vi "Work Paper No Record.vi"(8 "error in (no error)":errorcluster, 10 "Work No":refnum<vi>, 11 "Main Process Class in":refnum<class "Main Class.lvclass">) -> (0 "error out":errorcluster, 3 "Main Process Class out":refnum<class "Main Class.lvclass">)   [LabVIEW 2019]
uses:
  Main Class.lvclass
  Ctrl/Table Save.ctl
  LLB/Commonly VI/Main Glb.vi
  <vilib>/Utility/xml.llb/Write to XML File(string).vi
  LLB/Commonly VI.lvlib
panel:
  in  "Boolean":bool
  in  "Work No":string caption="工單號碼"
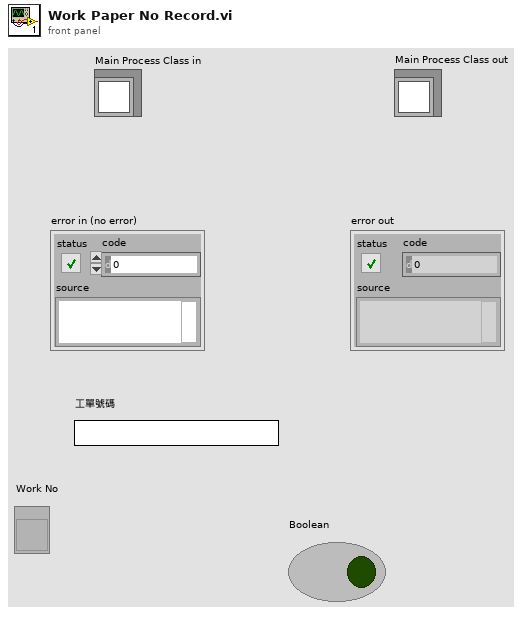
[diagram p1: front panel]
types:
  T1 = cluster{"AutoRunFlg":refnum<vi>, "Action Finish Flg":refnum<vi>, "Remaining Action":refnum<vi>, "Btn_AutoRun":refnum<vi>, "Manual Flg":refnum<vi>, "Sub Process Error":refnum<vi>}
  T2 = typedef "Table Save.ctl" = enum16{"initial", "Add", "Write", "Replace", "Delete", "REad", "RedTable", "Load"}
  T3 = typedef "工單號碼_Index.ctl" = enum16{"工單號碼", "產品料號", "品名", "作業員", "生產總數", "量品數量", "NG數量", "良率%"}
  T4 = cluster{"Work No":string, "產品料號":string, "品名":string, "Operator":string, "工單生產總數":string, "良品出料數量":string, "NG排出數量":string, "Total良率":string}
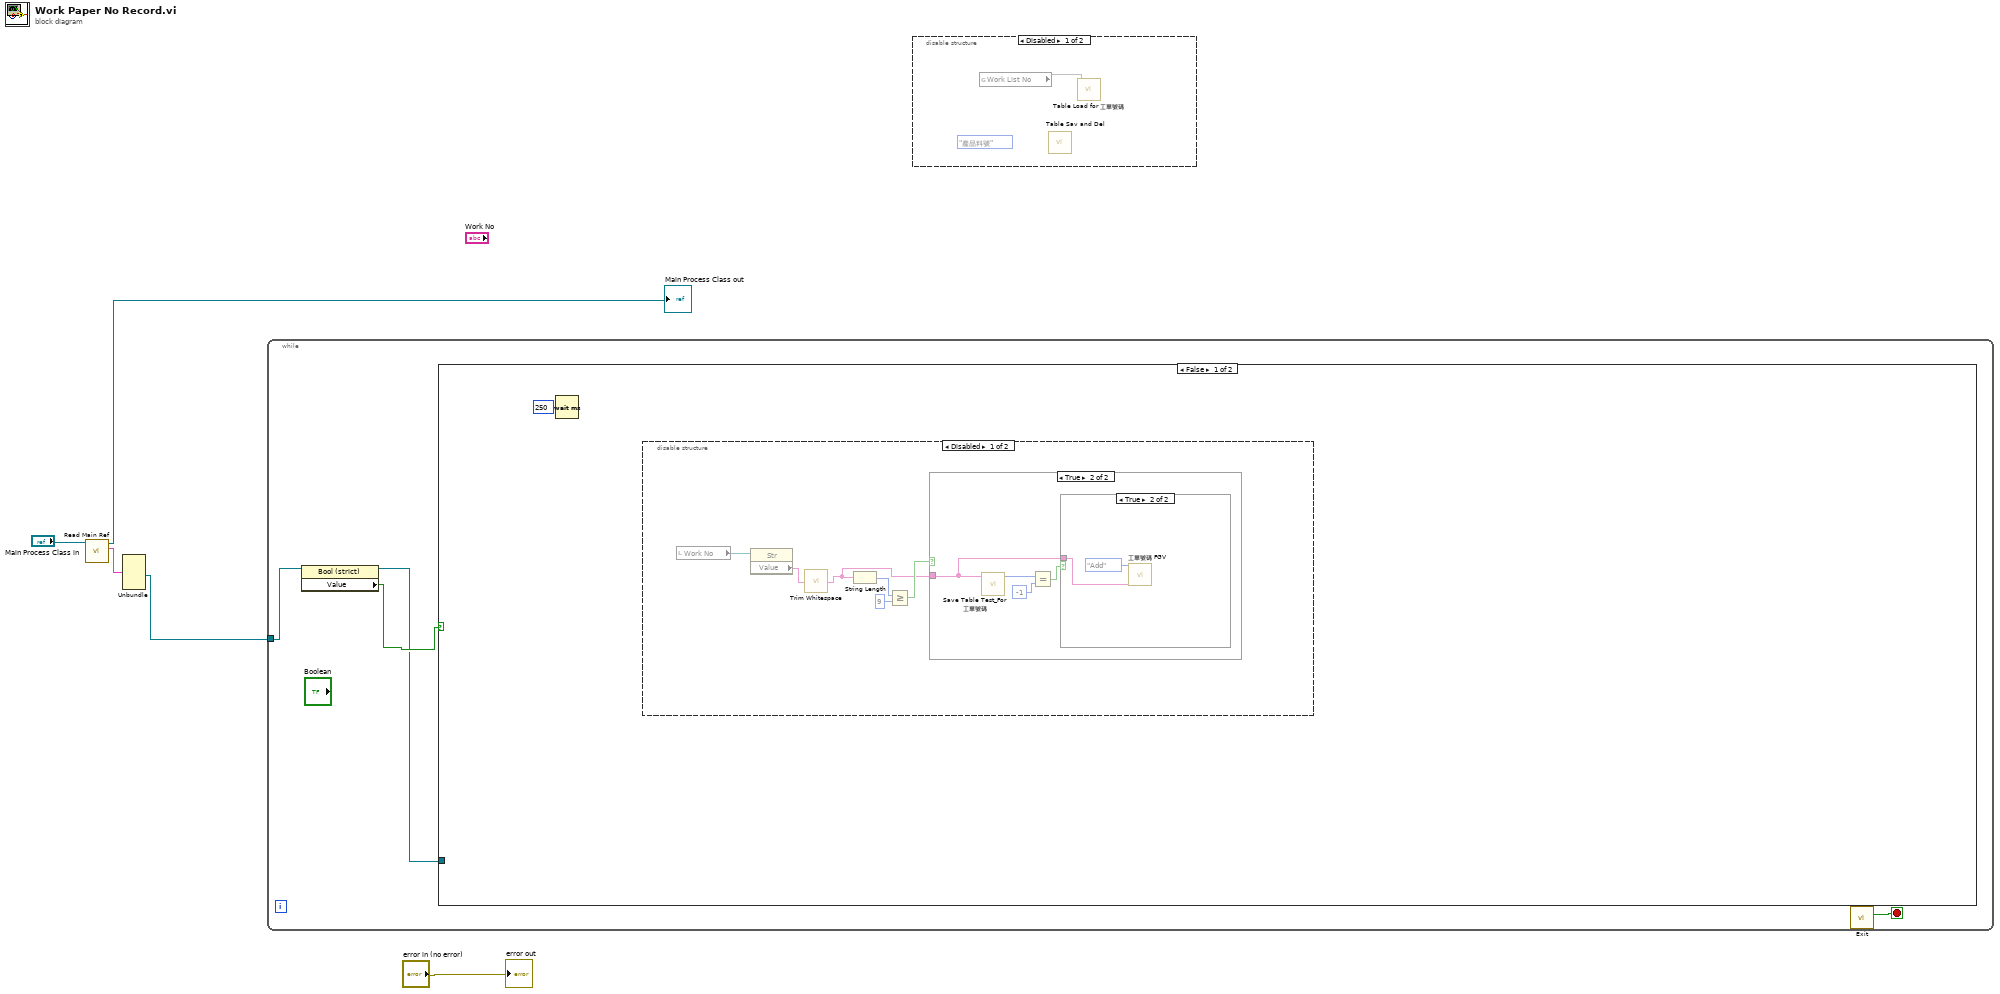
[diagram p0: block diagram]
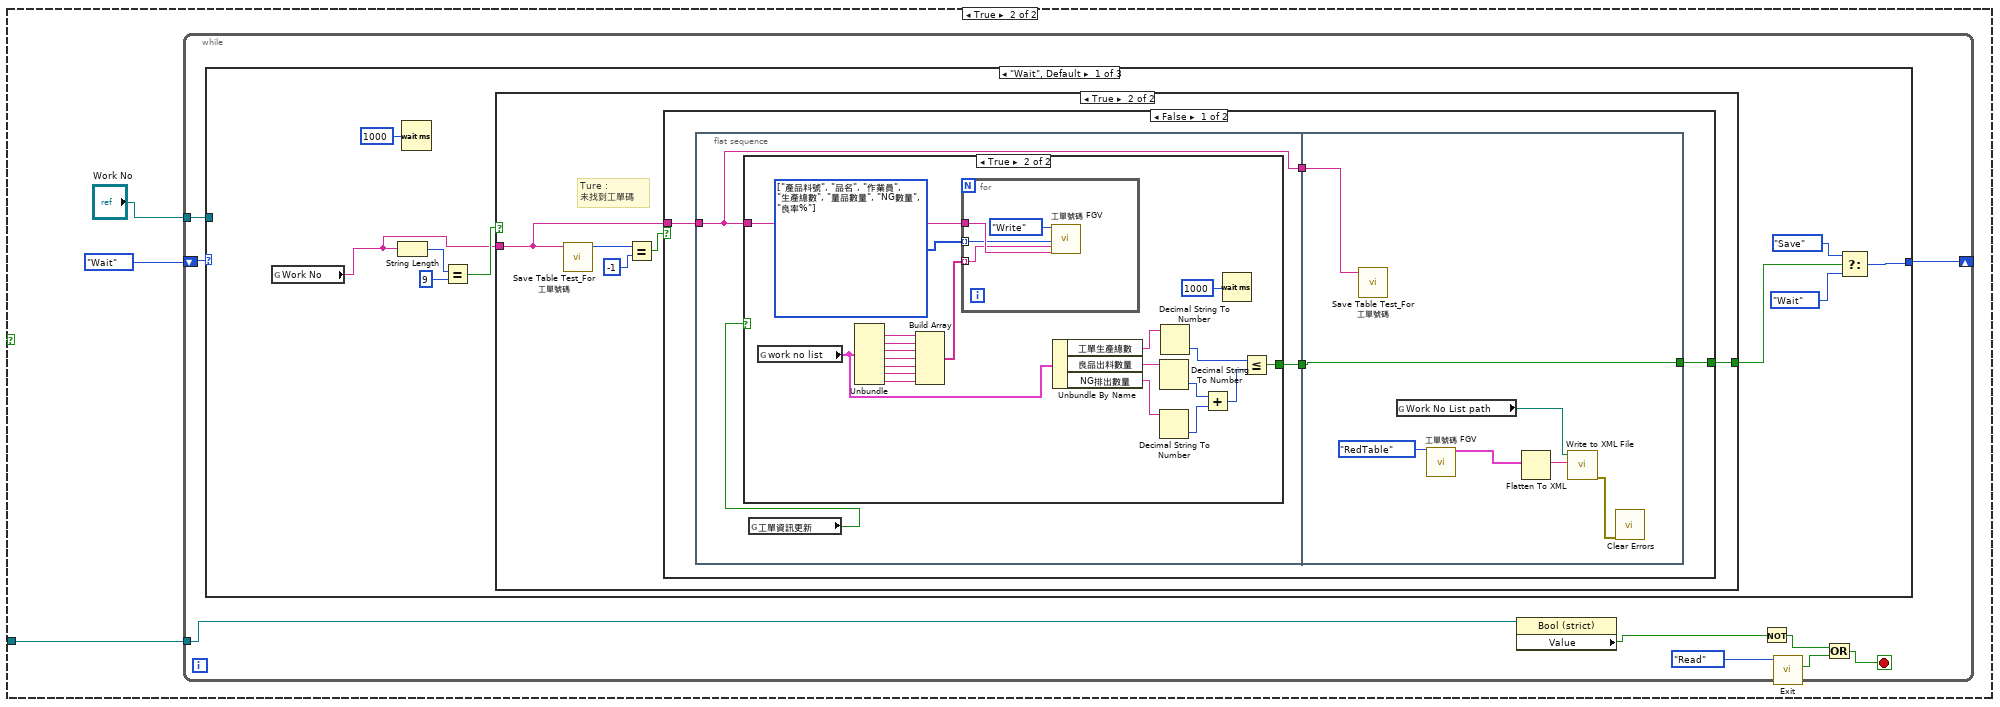
[diagram p6: hidden frame]
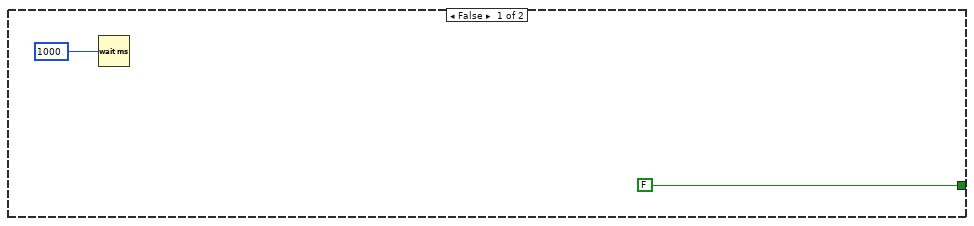
[diagram p7: hidden frame]
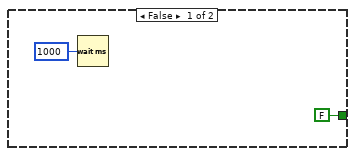
[diagram p8: hidden frame]
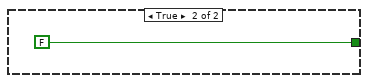
[diagram p9: hidden frame]
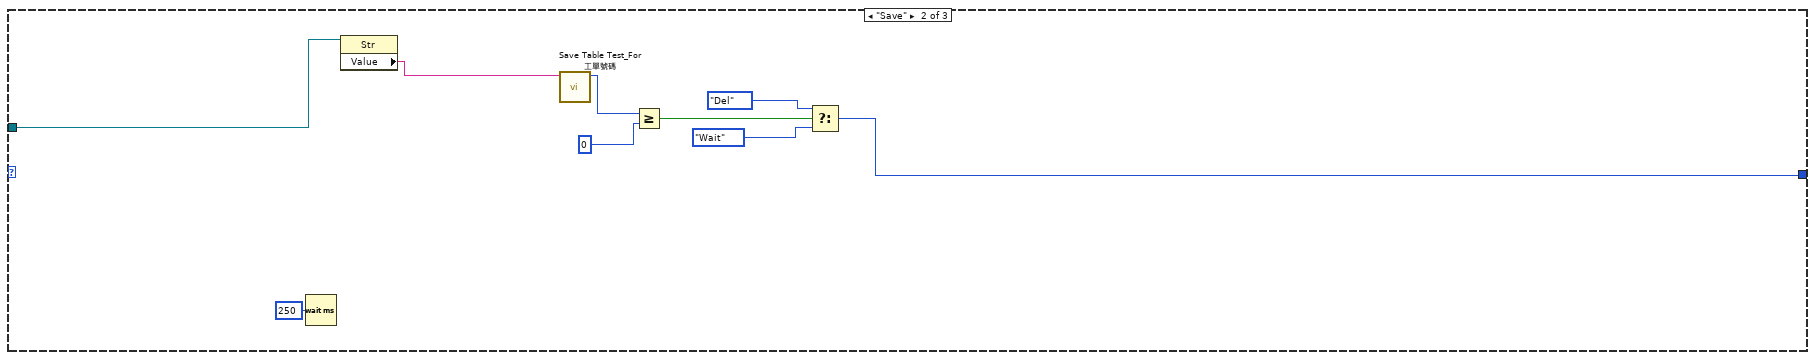
[diagram p10: hidden frame]
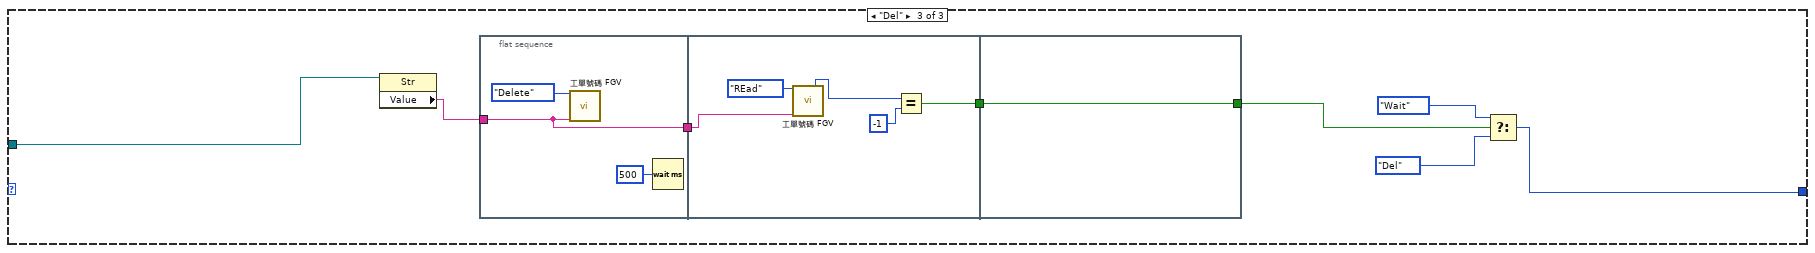
[diagram p11: hidden frame]
diagram:
  n1 = call-dynamic "Read Main Ref.vi"("Main Process Class in"="Main Process Class in") -> ("Main Ref"=w5:T1, "Main Process Class out"=→"Main Process Class out":refnum<class "Main Class.lvclass">)  [unwired: 8 in, 1 out]
  n2 = Unbundle(w5) -> ("Btn_AutoRun"=w2:refnum<vi>)  [unwired: 5 out]
  n3 = while {
    tunnel: w2 -> [w8]
    stop <- w9 stop-if-true
    n4 = property class="Bool (strict)"(reference=w8) -> (reference out=w6:refnum<vi>, "Value"=w7:bool)  [unwired: 1 in, 1 out]
    n5 = case shown="False" w7 {
      tunnel: w6 -> [_ w23]
      frame False {
        n6 = Wait (ms)(milliseconds to wait=u32 250) -> ()  [unwired: 1 out]
        n7 = disable-structure shown="Disabled" {
          frame Disabled {
            n8 = local read "Work No"() -> (w13:refnum<vi>)
            n9 = property class="Str"(reference=w13) -> ("Value"=w12:string)  [unwired: 1 in, 2 out]
            n10 = call <vilib>:"Trim Whitespace.vi"("string"=w12) -> ("trimmed string"=w11:string)  [unwired: 1 in]
            n11 = String Length(string=w11) -> (length=w16:i32)
            n12 = Greater Or Equal?(x=w16, y=9) -> (x >= y?=w14:bool)
            n13 = case shown="True" w14 {
              tunnel: w11 -> [_ w18]
              frame False {
              }
              frame True {
                n14 = call "Save Table Test_For 工單號碼.vi"("工單號碼"=w18) -> ("條碼的Index"=w19:i32)  [unwired: 9 in, 1 out]
                n15 = Equal?(x=w19, y=-1) -> (x = y?=w17:bool)
                n16 = case shown="True" w17 {
                  tunnel: w18 -> [_ w21]
                  frame False {
                  }
                  frame True {
                    n17 = call "工單號碼 FGV.vi"("Action"=Table_Save."Add", "工單號碼"=w21) -> ()  [unwired: 10 in, 8 out]
                  }
                }
              }
            }
          }
          frame Enabled {
          }
        }
      }
      frame True {
        n18 = while {
          shift-right: [w34] -> _
          shift-left: enum16{"Wait", "Save", "Del"}."Wait" -> [w33]
          tunnel: "Work No" -> [w32]
          tunnel: w23 -> [w27]
          stop <- w26 stop-if-true
          n19 = case shown="\"Wait\", Default" w33 {
            tunnel: [w37 w97 w102] -> w34
            tunnel: w32 -> [_ w96 w108]
            frame "Wait", Default {
              n20 = global read "Main Glb.vi" "Work No"() -> (w35:string)
              n21 = String Length(string=w35) -> (length=w42:i32)
              n22 = Wait (ms)(milliseconds to wait=u32 1000) -> ()  [unwired: 1 out]
              n23 = Equal?(x=w42, y=9) -> (x = y?=w40:bool)
              n24 = case shown="True" w40 {
                tunnel: w35 -> [_ w48]
                tunnel: [FALSE w46] -> w36
                frame False {
                  n25 = Wait (ms)(milliseconds to wait=u32 1000) -> ()  [unwired: 1 out]
                }
                frame True {
                  # "Ture : \n未找到工單碼"
                  n26 = call "Save Table Test_For 工單號碼.vi"("工單號碼"=w48) -> ("條碼的Index"=w49:i32)  [unwired: 9 in, 1 out]
                  n27 = Equal?(x=w49, y=-1) -> (x = y?=w47:bool)
                  n28 = case shown="False" w47 {
                    tunnel: w48 -> [w54 _]
                    tunnel: [w51 FALSE] -> w46
                    frame False {
                      n29 = flat-sequence {
                        tunnel: w54 -> [w57]
                        tunnel: [w57] -> w53
                        tunnel: [w56] -> w52
                        tunnel: w53 -> [w90]
                        tunnel: [w89] -> w51
                        tunnel: w52 -> [w89]
                        frame #0 {
                          n30 = global read "Main Glb.vi" "工單資訊更新"() -> (w55:bool)
                          n31 = case shown="True" w55 {
                            tunnel: w57 -> [_ w69]
                            tunnel: [FALSE w60] -> w56
                            frame False {
                              n32 = Wait (ms)(milliseconds to wait=u32 1000) -> ()  [unwired: 1 out]
                            }
                            frame True {
                              w79 = T3[] [enum."產品料號", enum."品名", enum."作業員", enum."生產總數", enum."量品數量", enum."NG數量", enum."良率%"] items=["工單號碼", "產品料號", "品名", "作業員", "生產總數", "量品數量", "NG數量", "良率%"]
                              n33 = global read "Main Glb.vi" "work no list"() -> (w70:T4)
                              n34 = Unbundle(w70) -> ("產品料號"=w78:string, "品名"=w77:string, "Operator"=w76:string, "工單生產總數"=w75:string, "良品出料數量"=w74:string, "NG排出數量"=w73:string, "Total良率"=w72:string)  [unwired: 1 out]
                              n35 = Build Array(w78, w77, w76, w75, w74, w73, w72) -> (w71:string[])
                              n36 = for {
                                tunnel: w69 -> [w82]
                                tunnel: w79 -> [w81] mode=indexing
                                tunnel: w71 -> [w80] mode=indexing
                                n37 = call "工單號碼 FGV.vi"("Action"=Table_Save."Write", "工單Data Save Index"=w81, "DataIn"=w80, "工單號碼"=w82) -> ()  [unwired: 8 in, 8 out]
                              }
                              n38 = Unbundle By Name(w70) -> ("工單生產總數"=w62:string, "良品出料數量"=w67:string, "NG排出數量"=w66:string)
                              n39 = Decimal String To Number(string=w67) -> (number=w65:i32)  [unwired: 2 in, 1 out]
                              n40 = Decimal String To Number(string=w66) -> (number=w64:i32)  [unwired: 2 in, 1 out]
                              n41 = Decimal String To Number(string=w62) -> (number=w61:i32)  [unwired: 2 in, 1 out]
                              n42 = Add(x=w65, y=w64) -> (x+y=w63:i32)
                              n43 = Wait (ms)(milliseconds to wait=u32 1000) -> ()  [unwired: 1 out]
                              n44 = Less Or Equal?(x=w61, y=w63) -> (x <= y?=w60:bool)
                            }
                          }
                        }
                        frame #1 {
                          n45 = call "Save Table Test_For 工單號碼.vi"("工單號碼"=w90) -> ()  [unwired: 9 in, 2 out]
                          n46 = global read "Main Glb.vi" "Work No List path"() -> (w88:path)
                          n47 = call "工單號碼 FGV.vi"("Action"=Table_Save."RedTable") -> ("Total Table"=w86:cluster{"Table Control":string[][]}[])  [unwired: 11 in, 7 out]
                          n48 = Flatten To XML(anything=w86) -> (xml string=w87:string)
                          n49 = call-poly <vilib>:"Write to XML File.vi"("XML Input"=w87, "XML File Path"=w88) -> ("error out"=w84:errorcluster)  [unwired: 7 in, 2 out]
                          n50 = call <vilib>:"Clear Errors.vi"("error in (no error)"=w84) -> ()  [unwired: 5 in, 2 out]
                        }
                      }
                    }
                    frame True {
                    }
                  }
                }
              }
              n51 = Select(t=enum16{"Wait", "Save", "Del"}."Save", s=w36, f=enum16{"Wait", "Save", "Del"}."Wait") -> (s? t:f=w37:enum16{"Wait", "Save", "Del"})
            }
            frame "Save" {
              n52 = Wait (ms)(milliseconds to wait=u32 250) -> ()  [unwired: 1 out]
              n53 = property class="Str"(reference=w96) -> ("Value"=w95:string)  [unwired: 1 in, 2 out]
              n54 = call "Save Table Test_For 工單號碼.vi"("工單號碼"=w95) -> ("條碼的Index"=w94:i32)  [unwired: 9 in, 1 out]
              n55 = Greater Or Equal?(x=w94, y=0) -> (x >= y?=w92:bool)
              n56 = Select(t=enum16{"Wait", "Save", "Del"}."Del", s=w92, f=enum16{"Wait", "Save", "Del"}."Wait") -> (s? t:f=w97:enum16{"Wait", "Save", "Del"})
            }
            frame "Del" {
              n57 = property class="Str"(reference=w108) -> ("Value"=w107:string)  [unwired: 1 in, 2 out]
              n58 = flat-sequence {
                tunnel: w107 -> [w110]
                tunnel: [w110] -> w106
                tunnel: w106 -> [w116]
                tunnel: [w112] -> w101
                tunnel: [w117] -> w103
                tunnel: w101 -> [w117]
                frame #0 {
                  n59 = call "工單號碼 FGV.vi"("Action"=Table_Save."Delete", "工單號碼"=w110) -> ()  [unwired: 10 in, 8 out]
                  n60 = Wait (ms)(milliseconds to wait=u32 500) -> ()  [unwired: 1 out]
                }
                frame #1 {
                  n61 = call "工單號碼 FGV.vi"("Action"=Table_Save."REad", "工單號碼"=w116) -> ("工單號碼的Index"=w113:i32)  [unwired: 10 in, 7 out]
                  n62 = Equal?(x=w113, y=-1) -> (x = y?=w112:bool)
                }
                frame #2 {
                }
              }
              n63 = Select(t=enum16{"Wait", "Save", "Del"}."Wait", s=w103, f=enum16{"Wait", "Save", "Del"}."Del") -> (s? t:f=w102:enum16{"Wait", "Save", "Del"})
            }
          }
          n64 = property class="Bool (strict)"(reference=w27) -> ("Value"=w29:bool)  [unwired: 1 in, 2 out]
          n65 = Not(x=w29) -> (.not. x?=w28:bool)
          n66 = call "Exit.vi"("Enum"=enum16{"Initial", "Read", "Write"}."Read") -> ("ExitOut"=w31:bool)  [unwired: 10 in]
          n67 = Or(x=w28, y=w31) -> (x .or. y?=w26:bool)
        }
      }
    }
    n68 = call "Exit.vi"() -> ("ExitOut"=w9:bool)  [unwired: 11 in]
  }
  n69 = disable-structure shown="Disabled" {
    frame Disabled {
      (unwired) 工單號碼_Index."產品料號" ("工單號碼Index")
      n70 = global read "Main Glb.vi" "Work List No"() -> (w118)
      n71 = call "Table Sav and Del.vi"() -> ()  [unwired: 10 in, 2 out]
      n72 = call "Table Load for 工單號碼.vi"("appended path"=w118) -> ()  [unwired: 10 in, 1 out]
    }
    frame Enabled {
    }
  }
  "error out" <- "error in (no error)"
